vi "xmlStringReadInt.vi"(3 "error in (no error)":errorcluster, 4 "String":string) -> (0 "error out":errorcluster, 1 "Value":i32)   [LabVIEW 2012]
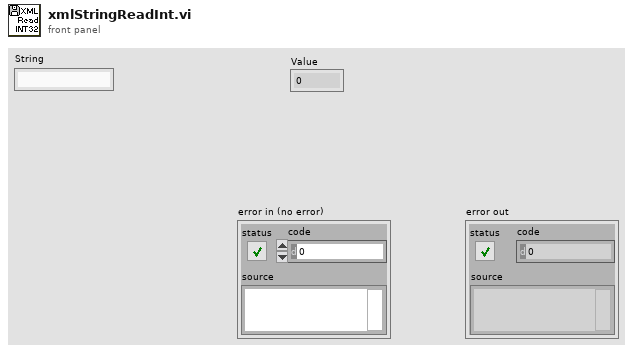
[diagram p1: front panel]
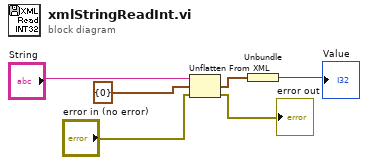
[diagram p0: block diagram]
diagram:
  n1 = Unflatten From XML(xml string="String", type=cluster{i32} {0}, error in (no error)="error in (no error)") -> (value=w5:cluster{i32}, error out=→"error out":errorcluster)
  n2 = Unbundle(w5) -> (→"Value":i32)
